vi "Get PPMS data.vi"(8 "error IO":errorcluster, 9 "control":string, 10 "Data Type":u16(ring) items=["String", "Double", "Boolean", "Variant"], 11 "vi reference":refnum<vi>) -> (0 "error out":errorcluster, 1 "Boolean":bool, 2 "Data (Double)":dbl format="%#_4g", 3 "Data (String)":string, 4 "vi reference out":refnum<vi>, 5 "Data (Variant)":variant)   [LabVIEW 2025]
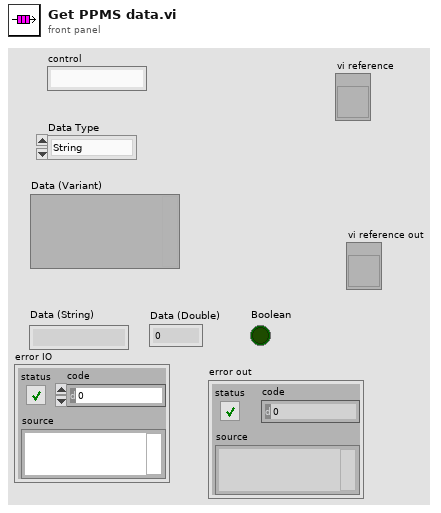
[diagram p1: front panel]
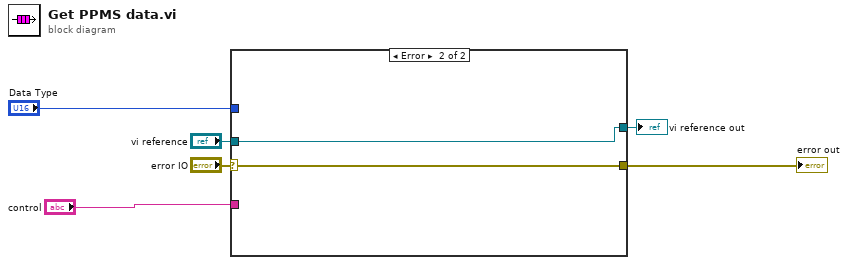
[diagram p0: block diagram]
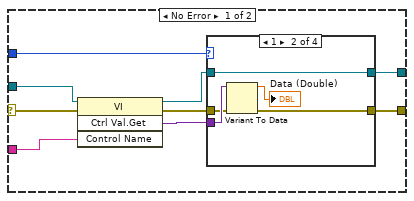
[diagram p2: hidden frame]
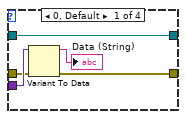
[diagram p3: hidden frame]
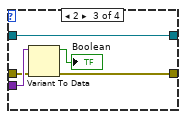
[diagram p4: hidden frame]
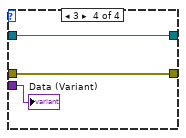
[diagram p5: hidden frame]
diagram:
  n1 = case shown="Error" "error IO" {
    selector: "error IO" -> [w11 w34]
    tunnel: "vi reference" -> [w15 w35]
    tunnel: [w10 w34] -> w1
    tunnel: [w9 w35] -> w2
    tunnel: "control" -> [w8 _]
    tunnel: "Data Type" -> [w7 _]
    frame No Error {
      n2 = invoke class="VI" method="Ctrl Val.Get"(reference=w15, error in=w11, "Control Name"=w8) -> (reference out=w12:refnum<vi>, error out=w13:errorcluster, "Get Control Value Variant"=w14:variant)  [unwired: 1 in, 1 out]
      n3 = case shown="1" w7 {
        tunnel: w14 -> [w20 w25 w30 w33]
        tunnel: w13 -> [w19 w24 w29 w32]
        tunnel: w12 -> [w16 w21 w26 w31]
        tunnel: [w17 w22 w27 w32] -> w10
        tunnel: [w16 w21 w26 w31] -> w9
        frame 0, Default {
          n4 = Variant To Data(error in=w19, Variant=w20) -> (data=→"Data (String)":string, error out=w17:errorcluster)  [unwired: 1 in]
        }
        frame 1 {
          n5 = Variant To Data(error in=w24, Variant=w25) -> (data=→"Data (Double)":dbl, error out=w22:errorcluster)  [unwired: 1 in]
        }
        frame 2 {
          n6 = Variant To Data(error in=w29, Variant=w30) -> (data=→"Boolean":bool, error out=w27:errorcluster)  [unwired: 1 in]
        }
        frame 3 {
          "Data (Variant)" <- w33
        }
      }
    }
    frame Error {
    }
  }
  "error out" <- w1
  "vi reference out" <- w2
